vi "Compute LO1 Frequency without Multiplication.vi"(8 "error in (no error)":errorcluster, 10 "Carrier Frequency":dbl format="%#_6p", 11 "Input LO1 Frequency":dbl format="%#_6p") -> (0 "error out":errorcluster, 3 "Output LO1 Frequency":dbl format="%#_6p")   [LabVIEW 2017]
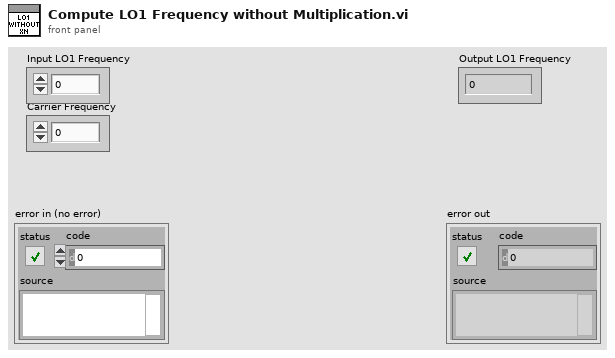
[diagram p1: front panel]
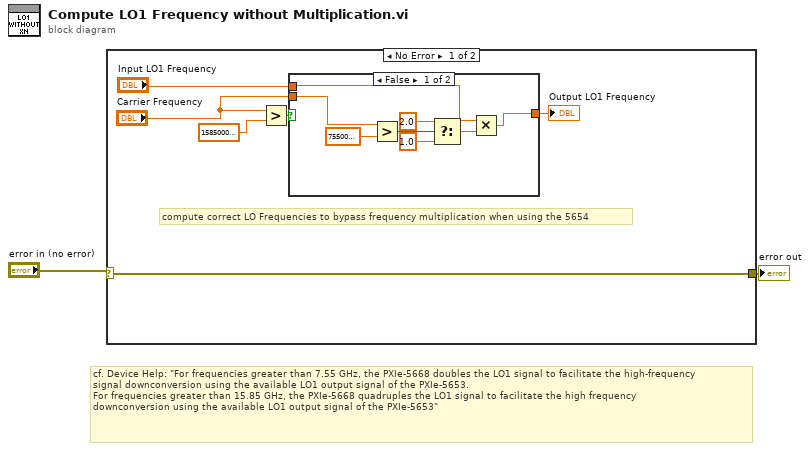
[diagram p0: block diagram]
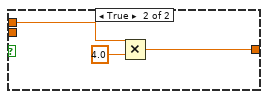
[diagram p2: hidden frame]
diagram:
  # "cf. Device Help: \"For frequencies greater than 7.55 GHz, the PXIe-5668 doubles the LO1 signal to facilitate the high-frequency \nsignal downconversion using the available LO1 output signal of the PXIe-5653. \nFor frequencies greater than 15.85 GHz, the PXIe-5668 quadruples the LO1 signal to facilitate the high frequency \ndownconversion using the available LO1 output signal of the PXIe-5653\""
  n1 = case shown="No Error" "error in (no error)" {
    selector: "error in (no error)" -> [w4 w20]
    tunnel: [w4 w20] -> w1
    frame No Error {
      # "compute correct LO Frequencies to bypass frequency multiplication when using the 5654"
      n2 = Greater?(x="Carrier Frequency", y=15850000000.0) -> (0:w7:bool)
      n3 = case shown="False" w7 {
        tunnel: "Carrier Frequency" -> [w11 _]
        tunnel: [w10 w18] -> w5
        tunnel: "Input LO1 Frequency" -> [w9 w17]
        frame False {
          n4 = Greater?(x=w11, y=7550000000.0) -> (0:w15:bool)
          n5 = Select(t=2.0, s=w15, f=1.0) -> (s? t:f=w12:dbl)
          n6 = Multiply(x=w9, y=w12) -> (x*y=w10:dbl)
        }
        frame True {
          n7 = Multiply(x=w17, y=4.0) -> (x*y=w18:dbl)
        }
      }
      "Output LO1 Frequency" <- w5
    }
    frame Error {
    }
  }
  "error out" <- w1
